vi "RSZVB Set Linearity Deviation Electrical Length.vi"(8 "error in (no error)":errorcluster {"code" format="%.0x"}, 9 "Electrical Length (0.0)":dbl format="%^.3e", 10 "Channel (1)":i32=1, 11 "VISA session":refnum<visa-resource-name>) -> (0 "error out":errorcluster {"code" format="%.0x"}, 3 "dup VISA session":refnum<visa-resource-name>)   [LabVIEW 2011]
doc: "This VI defines the electrical length for the linearity deviation calculation.\n\nNote(s):\n\n(1) Electrical length is available if the active trace format is Phase or Unwrapped Phase, or if a mixer delay is measured.\n\nRemote-control command(s):\nCALCulate<Chn>:LDEViation:ELENgth"
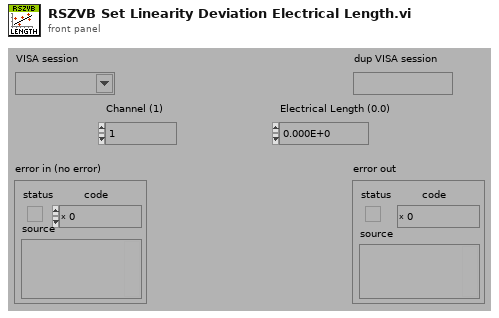
[diagram p1: front panel]
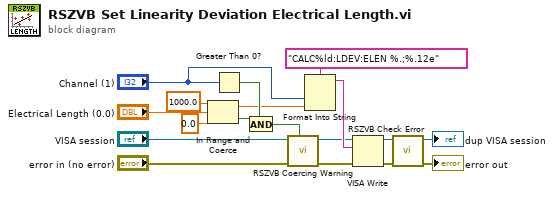
[diagram p0: block diagram]
diagram:
  n1 = In Range and Coerce(upper limit=1000.0, x="Electrical Length (0.0)", lower limit=0.0) -> (coerced(x)=w10:dbl, In Range?=w12:bool)
  n2 = Greater Than 0?(x="Channel (1)") -> (x > 0?=w11:bool)
  n3 = And(x=w11, y=w12) -> (x .and. y?=w13:bool)
  n4 = call "RSZVB Coercing Warning.vi"("In Range?"=w13, "error in (no error)"="error in (no error)", "VISA session"="VISA session") -> ("error out"=w9:errorcluster, "dup VISA session"=w14:refnum<visa-resource-name>)  [unwired: 7 in]
  n5 = Format Into String(format string="CALC%ld:LDEV:ELEN %.;%.12e", "Channel (1)", w10) -> (resulting string=w17:string)  [unwired: 2 in, 1 out]
  n6 = VISA Write(VISA resource name=w14, write buffer=w17, error in (no error)=w9) -> (VISA resource name out=w8:refnum<visa-resource-name>, error out=w7:errorcluster)  [unwired: 1 out]
  n7 = call "RSZVB Check Error.vi"("error in (no error)"=w7, "VISA session"=w8) -> ("error out"=→"error out":errorcluster, "dup VISA session"=→"dup VISA session":refnum<visa-resource-name>)  [unwired: 8 in]
